vi "DTbl Analog to Digital.vi"(6 "data format (offset binary)":u16(ring)=1 items=["unsigned binary", "offset binary", "2's complement"], 7 "compress digital (T)":bool=TRUE, 8 "error in (no error)":errorcluster, 9 "full-scale range (pk-pk)":dbl=2.0 caption="full scale range (pk-pk)", 10 "resolution (16 bit)":i32=16, 11 "analog waveform":waveform(dbl)) -> (0 "error out":errorcluster, 1 "full-scale range (out)":dbl=2.0, 2 "resolution (out)":i32=16, 3 "digital data":digitaldata)   [LabVIEW 2020]
doc: "Converts <B>analog waveform</B> to a digital waveform or digital data. You must manually select the polymorphic instance you want to use."
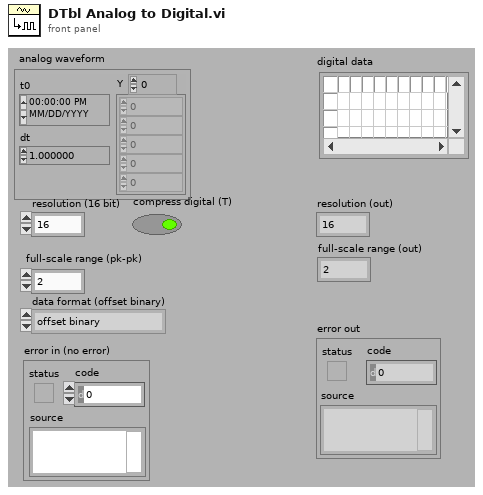
[diagram p1: front panel]
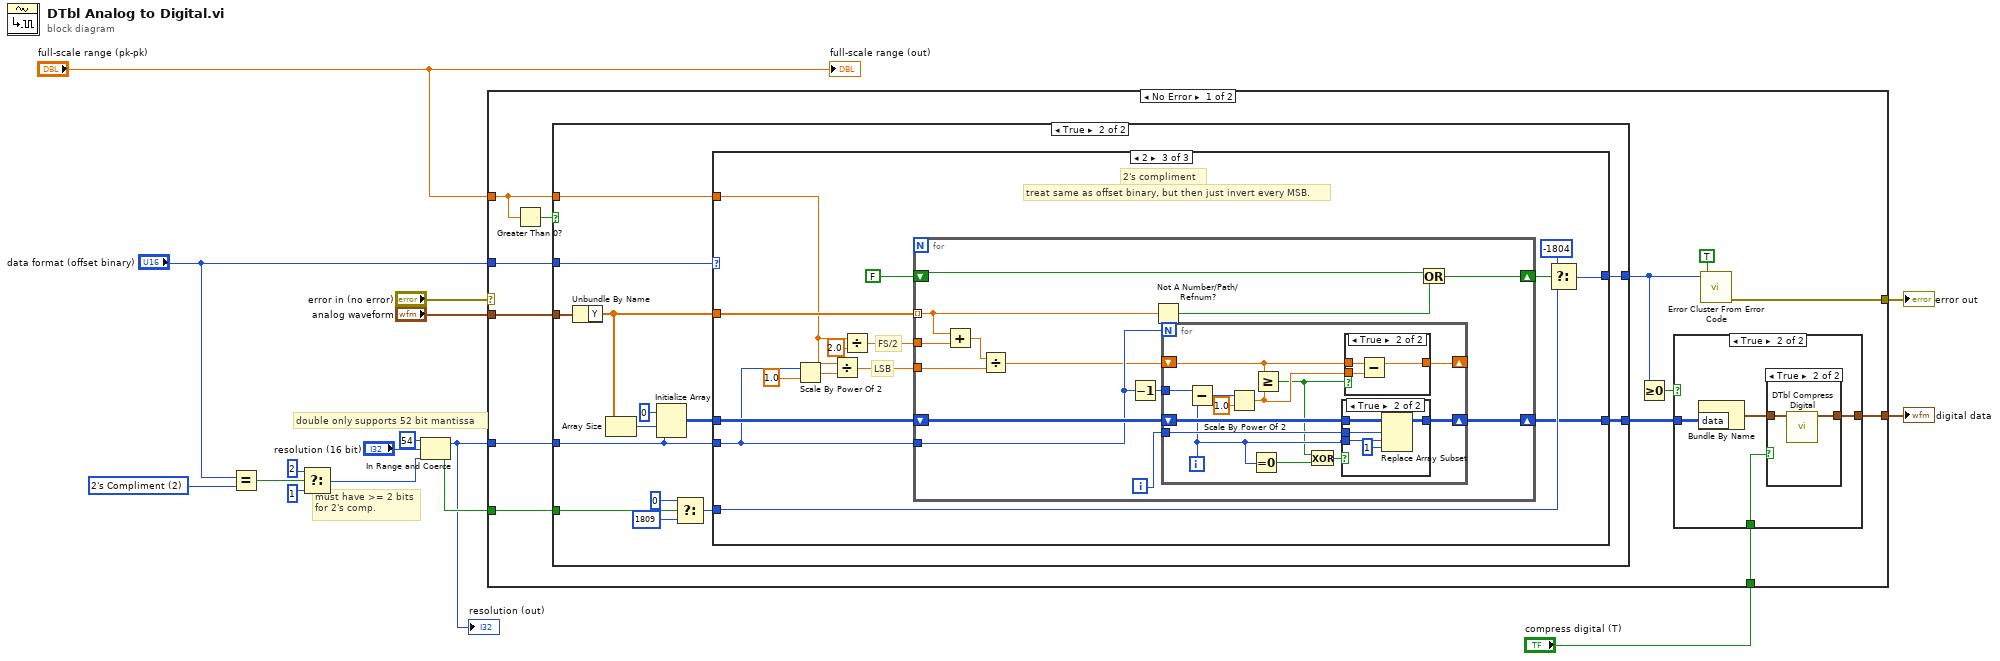
[diagram p0: block diagram]
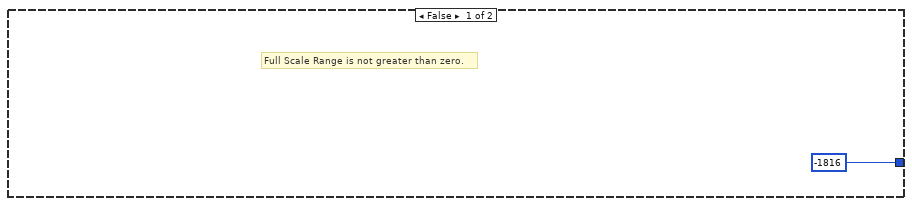
[diagram p2: hidden frame]
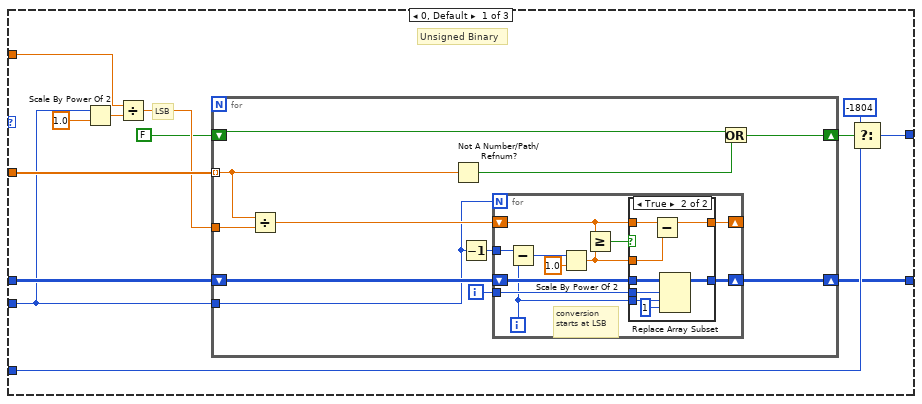
[diagram p3: hidden frame]
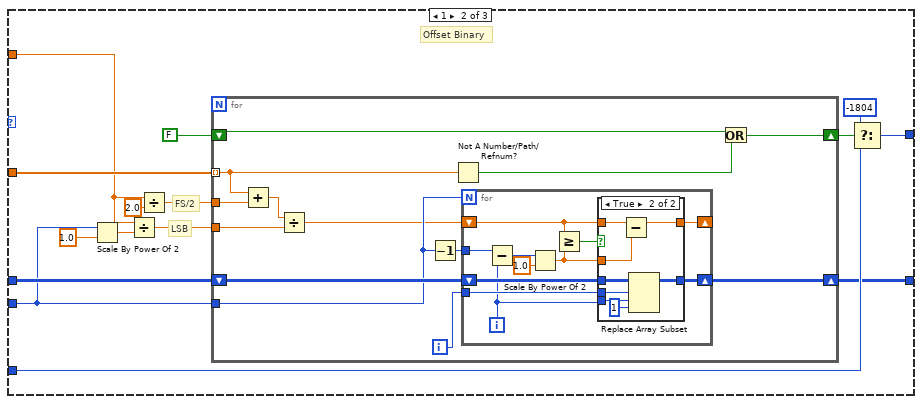
[diagram p5: hidden frame]
diagram:
  w1 = u16 2 items=["Unsigned Binary", "Offset Binary", "2's Compliment"] ("data format (offset binary)")
  # "must have >= 2 bits\nfor 2's comp."
  # "double only supports 52 bit mantissa"
  n1 = Equal?(x="data format (offset binary)", y=w1) -> (x = y?=w2:bool)
  n2 = Select(t=2 ("lower limit"), s=w2, f=1 ("lower limit")) -> (s? t:f=w6:i32)
  n3 = In Range and Coerce(upper limit=54, x="resolution (16 bit)", lower limit=w6) -> (coerced(x)=w10:i32, In Range?=w11:bool)
  "resolution (out)" <- w10
  n4 = case shown="No Error" "error in (no error)" {
    selector: "error in (no error)" -> [_ w197]
    tunnel: "analog waveform" -> [w29 _]
    tunnel: [w24 _] -> w5
    tunnel: w10 -> [w27 _]
    tunnel: [w20 w197] -> w12
    tunnel: w11 -> [w28 _]
    tunnel: "full-scale range (pk-pk)" -> [w18 _]
    tunnel: "compress digital (T)" -> [w23 _]
    tunnel: "data format (offset binary)" -> [w22 _]
    frame No Error {
      n5 = Greater Than 0?(x=w18) -> (x > 0?=w17:bool)
      n6 = case shown="True" w17 {
        tunnel: w29 -> [_ w44]
        tunnel: w28 -> [_ w41]
        tunnel: w27 -> [_ w37]
        tunnel: [_ w34] -> w26
        tunnel: w22 -> [_ w33]
        tunnel: [-1816 ("f") w32] -> w21
        tunnel: w18 -> [_ w31]
        frame False {
          # "Full Scale Range is not greater than zero."
        }
        frame True {
          n7 = Unbundle By Name(w44) -> ("Y"=w36:dbl[])
          n8 = Array Size(array=w36) -> (size(s)=w40:i32)
          n9 = Initialize Array(u8 0, w40, w37) -> (w38:u8[][])
          n10 = Select(t=0, s=w41, f=1809) -> (s? t:f=w35:i32)
          n11 = case shown="2" w33 {
            tunnel: w31 -> [w45 w93 w142]
            tunnel: w38 -> [w57 w104 w153]
            tunnel: w36 -> [w56 w103 w152]
            tunnel: w37 -> [w47 w90 w139]
            tunnel: w35 -> [w51 w99 w148]
            tunnel: [w50 w98 w147] -> w34
            tunnel: [w49 w97 w146] -> w32
            frame 0, Default {
              # "Unsigned Binary"
              # "LSB"
              n12 = Scale By Power Of 2(n=w47, x=1.0) -> (x*2^n=w46:dbl)
              n13 = Divide(x=w45, y=w46) -> (x/y=w55:dbl)
              n14 = for {
                shift-right: [w66] -> w50
                shift-left: w57 -> [w67]
                tunnel: w56 -> [w58] mode=indexing
                tunnel: w55 -> [w63]
                shift-right: [w64] -> w53
                shift-left: FALSE ("f") -> [w60]
                tunnel: w47 -> [w62]
                i -> [w65]
                n15 = Divide(x=w58, y=w63) -> (x/y=w68:dbl)
                n16 = Not A Number/Path/Refnum?(number/path/refnum=w58) -> (NaN/Path/Refnum?=w59:bool)
                n17 = Decrement(x=w62) -> (x-1=w61:i32)
                n18 = for {
                  N: w62 -> [_]
                  shift-right: [w73] -> _
                  shift-left: w68 -> [w74]
                  tunnel: w61 -> [w79]
                  shift-right: [w76] -> w66
                  shift-left: w67 -> [w77]
                  tunnel: w65 -> [w75]
                  i -> [w69]
                  # "conversion \nstarts at LSB"
                  n19 = Subtract(x=w79, y=w69) -> (x-y=w70:i32)
                  n20 = Scale By Power Of 2(n=w70, x=1.0) -> (x*2^n=w71:dbl)
                  n21 = Greater Or Equal?(x=w74, y=w71) -> (x >= y?=w78:bool)
                  n22 = case shown="True" w78 {
                    tunnel: w77 -> [w80 w89]
                    tunnel: [w80 w88] -> w76
                    tunnel: w69 -> [_ w87]
                    tunnel: w75 -> [_ w86]
                    tunnel: w74 -> [w81 w84]
                    tunnel: w71 -> [_ w83]
                    tunnel: [w81 w82] -> w73
                    frame False {
                    }
                    frame True {
                      n23 = Subtract(x=w84, y=w83) -> (x-y=w82:dbl)
                      n24 = Replace Array Subset(array=w89, new element=u8 1 ("New Element/Subarray"), index (row)=w86, index (col)=w87) -> (w88:u8[][])
                    }
                  }
                }
                n25 = Or(x=w60, y=w59) -> (x .or. y?=w64:bool)
              }
              n26 = Select(t=-1804, s=w53, f=w51) -> (s? t:f=w49:i32)
            }
            frame 1 {
              # "FS/2"
              # "LSB"
              # "Offset Binary"
              n27 = Scale By Power Of 2(n=w90, x=1.0) -> (x*2^n=w95:dbl)
              n28 = Divide(x=w93, y=w95) -> (x/y=w94:dbl)
              n29 = Divide(x=w93, y=2.0) -> (x/y=w91:dbl)
              n30 = for {
                shift-right: [w105] -> w98
                shift-left: w104 -> [w117]
                tunnel: w103 -> [w109] mode=indexing
                tunnel: w94 -> [w108]
                shift-right: [w116] -> w101
                shift-left: FALSE ("f") -> [w114]
                tunnel: w90 -> [w111]
                tunnel: w91 -> [w110]
                i -> [w112]
                n31 = Add(x=w109, y=w110) -> (x+y=w107:dbl)
                n32 = Divide(x=w107, y=w108) -> (x/y=w106:dbl)
                n33 = Decrement(x=w111) -> (x-1=w115:i32)
                n34 = Not A Number/Path/Refnum?(number/path/refnum=w109) -> (NaN/Path/Refnum?=w113:bool)
                n35 = for {
                  N: w111 -> [_]
                  shift-right: [w122] -> _
                  shift-left: w106 -> [w123]
                  tunnel: w115 -> [w128]
                  shift-right: [w125] -> w105
                  shift-left: w117 -> [w126]
                  tunnel: w112 -> [w124]
                  i -> [w118]
                  n36 = Subtract(x=w128, y=w118) -> (x-y=w119:i32)
                  n37 = Scale By Power Of 2(n=w119, x=1.0) -> (x*2^n=w120:dbl)
                  n38 = Greater Or Equal?(x=w123, y=w120) -> (x >= y?=w127:bool)
                  n39 = case shown="True" w127 {
                    tunnel: w126 -> [w129 w138]
                    tunnel: [w129 w137] -> w125
                    tunnel: w118 -> [_ w136]
                    tunnel: w124 -> [_ w135]
                    tunnel: w123 -> [w130 w133]
                    tunnel: w120 -> [_ w132]
                    tunnel: [w130 w131] -> w122
                    frame False {
                    }
                    frame True {
                      n40 = Subtract(x=w133, y=w132) -> (x-y=w131:dbl)
                      n41 = Replace Array Subset(array=w138, new element=u8 1 ("New Element/Subarray"), index (row)=w135, index (col)=w136) -> (w137:u8[][])
                    }
                  }
                }
                n42 = Or(x=w114, y=w113) -> (x .or. y?=w116:bool)
              }
              n43 = Select(t=-1804, s=w101, f=w99) -> (s? t:f=w97:i32)
            }
            frame 2 {
              # "treat same as offset binary, but then just invert every MSB."
              # "FS/2"
              # "LSB"
              # "2's compliment"
              n44 = Scale By Power Of 2(n=w139, x=1.0) -> (x*2^n=w144:dbl)
              n45 = Divide(x=w142, y=w144) -> (x/y=w143:dbl)
              n46 = Divide(x=w142, y=2.0) -> (x/y=w140:dbl)
              n47 = for {
                shift-right: [w154] -> w147
                shift-left: w153 -> [w166]
                tunnel: w152 -> [w158] mode=indexing
                tunnel: w143 -> [w157]
                shift-right: [w165] -> w150
                shift-left: FALSE ("f") -> [w163]
                tunnel: w139 -> [w160]
                tunnel: w140 -> [w159]
                i -> [w161]
                n48 = Add(x=w158, y=w159) -> (x+y=w156:dbl)
                n49 = Divide(x=w156, y=w157) -> (x/y=w155:dbl)
                n50 = Decrement(x=w160) -> (x-1=w164:i32)
                n51 = Not A Number/Path/Refnum?(number/path/refnum=w158) -> (NaN/Path/Refnum?=w162:bool)
                n52 = for {
                  N: w160 -> [_]
                  shift-right: [w174] -> _
                  shift-left: w155 -> [w175]
                  tunnel: w164 -> [w179]
                  shift-right: [w177] -> w154
                  shift-left: w166 -> [w178]
                  tunnel: w161 -> [w176]
                  i -> [w169]
                  n53 = Subtract(x=w179, y=w169) -> (x-y=w170:i32)
                  n54 = Scale By Power Of 2(n=w170, x=1.0) -> (x*2^n=w172:dbl)
                  n55 = Equal To 0?(x=w169) -> (x = 0?=w171:bool)
                  n56 = Greater Or Equal?(x=w175, y=w172) -> (x >= y?=w168:bool)
                  n57 = Exclusive Or(1:w171, 2:w168) -> (0:w167:bool)
                  n58 = case shown="True" w167 {
                    tunnel: w178 -> [w180 w185]
                    tunnel: [w180 w184] -> w177
                    tunnel: w176 -> [_ w183]
                    tunnel: w169 -> [_ w182]
                    frame False {
                    }
                    frame True {
                      n59 = Replace Array Subset(array=w185, new element=u8 1 ("New Element/Subarray"), index (row)=w183, index (col)=w182) -> (w184:u8[][])
                    }
                  }
                  n60 = case shown="True" w168 {
                    tunnel: w175 -> [w186 w189]
                    tunnel: [w186 w188] -> w174
                    tunnel: w172 -> [_ w187]
                    frame False {
                    }
                    frame True {
                      n61 = Subtract(x=w189, y=w187) -> (x-y=w188:dbl)
                    }
                  }
                }
                n62 = Or(x=w163, y=w162) -> (x .or. y?=w165:bool)
              }
              n63 = Select(t=-1804, s=w150, f=w148) -> (s? t:f=w146:i32)
            }
          }
        }
      }
      n64 = Greater Or Equal To 0?(x=w21) -> (x >= 0?=w25:bool)
      n65 = case shown="True" w25 {
        tunnel: [_ w193] -> w24
        tunnel: w26 -> [_ w191]
        tunnel: w23 -> [_ w190]
        frame False {
        }
        frame True {
          n66 = Bundle By Name("data"=w191) -> (w192:digitaldata)  [unwired: 1 in]
          n67 = case shown="True" w190 {
            tunnel: [w194 w196] -> w193
            tunnel: w192 -> [w194 w195]
            frame False {
            }
            frame True {
              n68 = call "DTbl Compress Digital.vi"("uncompressed digital data"=w195) -> ("compressed digital data"=w196:digitaldata)  [unwired: 9 in, 1 out]
            }
          }
        }
      }
      n69 = call "Error Cluster From Error Code.vi"("show call chain? (False)"=TRUE, "error code (0)"=w21) -> ("error out"=w20:errorcluster)  [unwired: 7 in]
    }
    frame Error {
      # "Return empty array\non input error."
    }
  }
  "error out" <- w12
  "digital data" <- w5
  "full-scale range (out)" <- "full-scale range (pk-pk)"
